vi "XY  Graph Get Multiple Scales Information.vi"(8 "error in (no error)":errorcluster, 9 "X(F)/Y(T)":bool, 10 "[Scale Idx]":u32[](array[numeric]), 11 "XYGraph Ref":refnum<vi>) -> (0 "error out":errorcluster, 3 "[Scale Information]":T1)   [LabVIEW 2021, in "XY Graph Add-Ons.lvlib"]
uses:
  XY Graph Add-Ons.lvlib
  Graph Scale Information.ctl
  Graphs.lvlib
  XY Graph Scales Information.ctl
panel:
  # "see the License on the block diagram (Ctrl+E or Window:Show Block Diagram)"
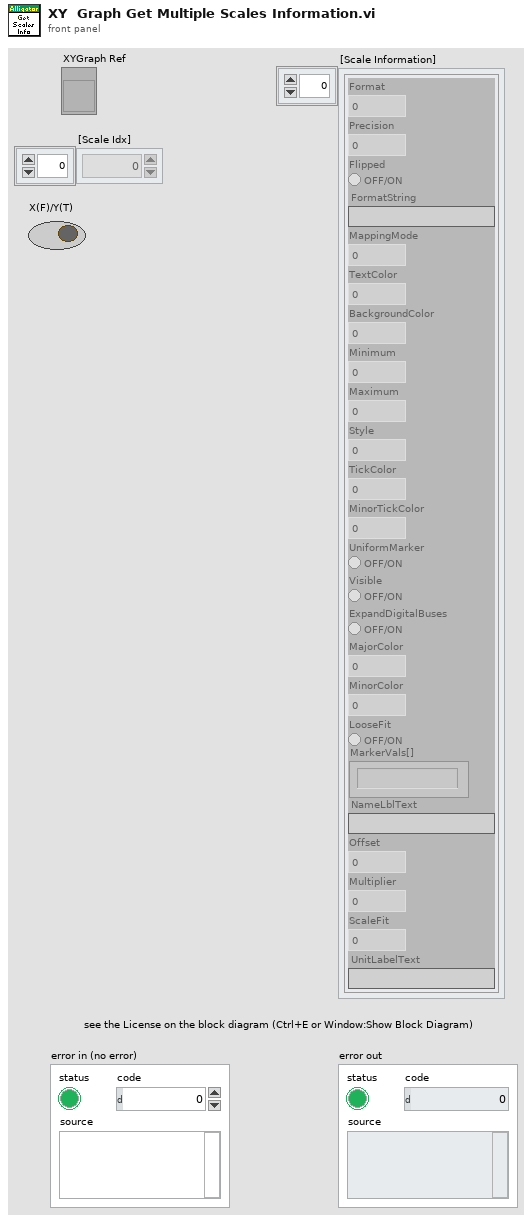
[diagram p1: front panel]
types:
  T1 = typedef "XY Graph Add-Ons.lvlib/XY Graph Scales Information.ctl" = T2[]
  T2 = typedef "Graphs.lvlib/Graph Scale Information.ctl" = cluster{"Format":u8, "Precision":u8, "Flipped":bool, "FormatString":string, "MappingMode":u8, "TextColor":u32, "BackgroundColor":u32, "Minimum":dbl, "Maximum":dbl, "Style":u8, "TickColor":u32, "MinorTickColor":u32, "UniformMarker":bool, "Visible":bool, "ExpandDigitalBuses":bool, "MajorColor":u32, "MinorColor":u32, "LooseFit":bool, "MarkerVals[]":string, "NameLblText":string, "Offset":dbl, "Multiplier":dbl, "ScaleFit":u8, "UnitLabelText":string}
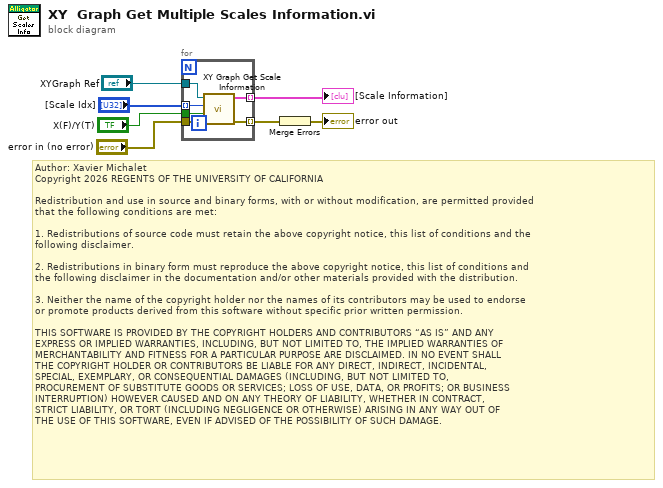
[diagram p0: block diagram]
diagram:
  # "Author: Xavier Michalet\nCopyright 2026 REGENTS OF THE UNIVERSITY OF CALIFORNIA\n\nRedistribution and use in source and binary forms, with or without modification, are permitted provided\nthat the following conditions are met:\n\n1. Redistributions of source code must retain the above copyright notice, this list of conditions and the\nfollowing disclaimer.\n\n2. Redistributions in binary form must reproduce the above copyright notice, this list of conditions and\nthe following disclaimer in the documentation and/or other materials provided with the distribution.\n\n3. Neither the name of the copyright holder nor the names of its contributors may be used to endorse \nor promote products derived from this software without specific prior written permission.\n\nTHIS SOFTWARE IS PROVIDED BY THE COPYRIGHT HOLDERS AND CONTRIBUTORS “AS IS” AND ANY \nEXPRESS OR IMPLIED WARRANTIES, INCLUDING, BUT NOT LIMITED TO, THE IMPLIED WARRANTIES OF\nMERCHANTABILITY AND FITNESS FOR A PARTICULAR PURPOSE ARE DISCLAIMED. IN NO EVENT SHALL\nTHE COPYRIGHT HOLDER OR CONTRIBUTORS BE LIABLE FOR ANY DIRECT, INDIRECT, INCIDENTAL, \nSPECIAL, EXEMPLARY, OR CONSEQUENTIAL DAMAGES (INCLUDING, BUT NOT LIMITED TO, \nPROCUREMENT OF SUBSTITUTE GOODS OR SERVICES; LOSS OF USE, DATA, OR PROFITS; OR BUSINESS\nINTERRUPTION) HOWEVER CAUSED AND ON ANY THEORY OF LIABILITY, WHETHER IN CONTRACT, \nSTRICT LIABILITY, OR TORT (INCLUDING NEGLIGENCE OR OTHERWISE) ARISING IN ANY WAY OUT OF\nTHE USE OF THIS SOFTWARE, EVEN IF ADVISED OF THE POSSIBILITY OF SUCH DAMAGE."
  n1 = for {
    tunnel: "[Scale Idx]" -> [w13] mode=indexing
    tunnel: [w12] -> w5 mode=indexing
    tunnel: [w11] -> w6 mode=indexing
    tunnel: "error in (no error)" -> [w10]
    tunnel: "XYGraph Ref" -> [w9]
    tunnel: "X(F)/Y(T)" -> [w8]
    n2 = call "XY Graph Get Scale Information.vi"("error in (no error)"=w10, "X(F)/Y(T)"=w8, "Plot.ScaleIdx"=w13, "XYGraph Ref"=w9) -> ("Error Out"=w11:errorcluster, "Graph Scale Information"=w12:T2)  [unwired: 6 in]
  }
  "[Scale Information]" <- w5
  n3 = Merge Errors(w6) -> (→"error out":errorcluster)
